vi "SCTL Sector Accumulation V2.vi"() -> (3 "New Data?":bool)   [LabVIEW 2013]
uses:
  <vilib>/rvi/Memory/Memory_Emulation/niFpgaMemoryEmulationReadFromVariant.vi
  <vilib>/rvi/Emulation/niFpgaSctlEmulationGetInTimedLoop.vi
  <vilib>/rvi/Memory/Memory_Emulation/niFpgaMemoryEmulationWriteToVariant.vi
  <vilib>/rvi/DataTransferAndStorage/Container/Common/niFpgaContainerGetUniqueNameForEmu.vi
  <vilib>/rvi/FIFO/Fifo_Resource/nirvififoEmulationSetSize.vi
  <vilib>/rvi/Emulation/niFpgaSctlEmulationFifoFullMgr.vi
  <vilib>/rvi/errors/niFpgaSetErrorForExecOnDevCompSimple.vi
  <vilib>/rvi/eio/common/nirviEmuReportErrorAndStop.vi
  <vilib>/rvi/Emulation/niFpgaSctlEmulationResourceMgr.vi
  <vilib>/rvi/Memory/Memory_Emulation/nirvimemoryFastEmulation.vi
  <vilib>/rvi/Memory/Memory_Emulation/nirvimemoryEmulation.vi
  <vilib>/rvi/DataTransferAndStorage/Container/XNode/niFpgaContainer.xnode
  <vilib>/rvi/FIFO/Fifo_Resource/nirvififoEmulationRead.vi
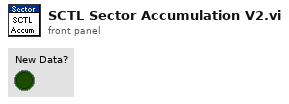
[diagram p1: front panel]
types:
  T1 = cluster{"Accumulated Intensity":u32, "Count":u16}
  T2 = cluster{"Accumulated Intensity":u32, "Count":u16}[]
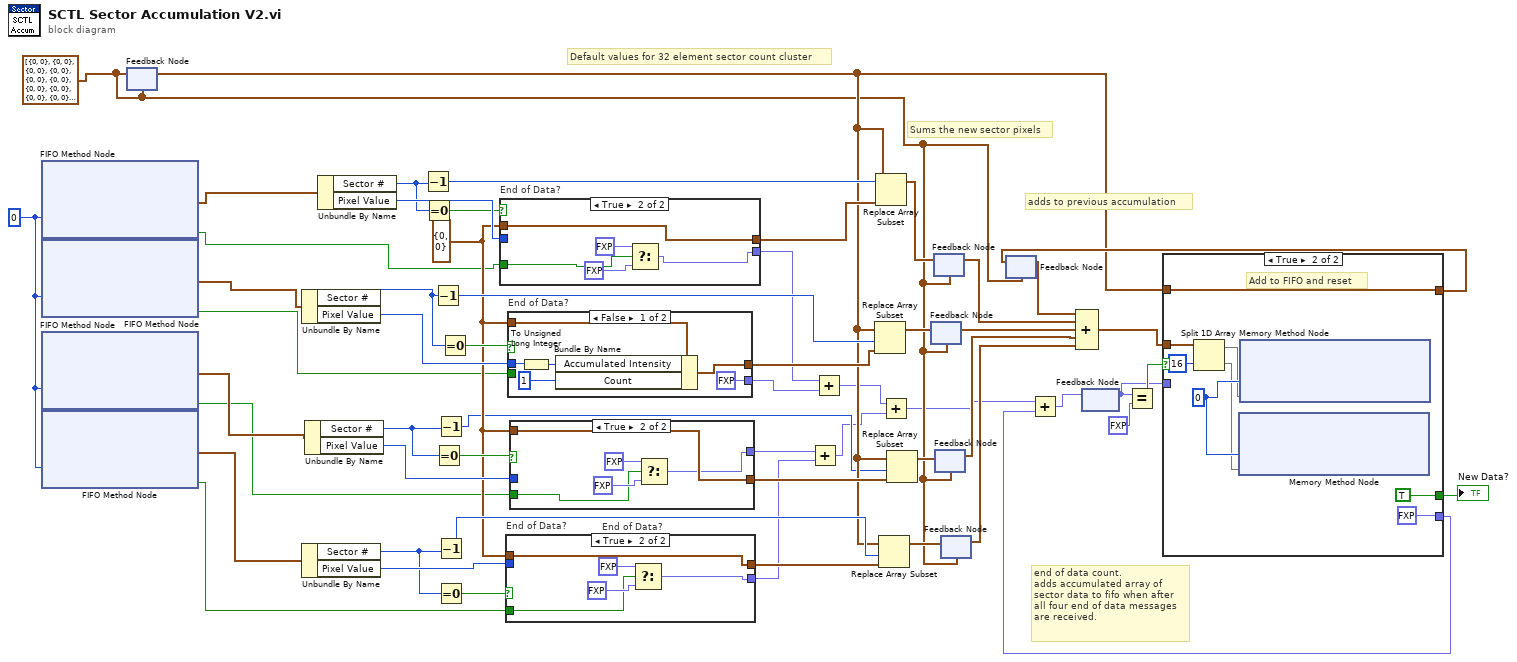
[diagram p0: block diagram]
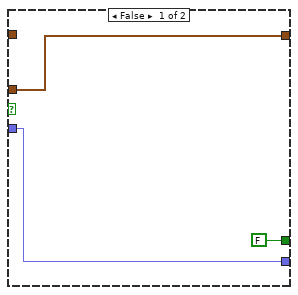
[diagram p2: hidden frame]
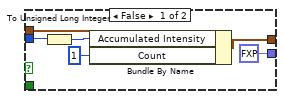
[diagram p3: hidden frame]
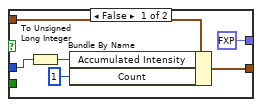
[diagram p4: hidden frame]
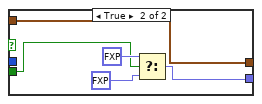
[diagram p5: hidden frame]
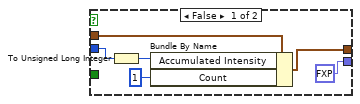
[diagram p6: hidden frame]
diagram:
  w32 = T1 {"Accumulated Intensity"=0, "Count"=0} ("Accumulated Sector Cluster")
  w10 = T2 [{"Accumulated Intensity"=0, "Count"=0}, {"Accumulated Intensity"=0, "Count"=0}, {"Accumulated Intensity"=0, "Count"=0}, {"Accumulated Intensity"=0, "Count"=0}, {"Accumulated Intensity"=0, "Count"=0}, {"Accumulated Intensity"=0, "Count"=0}, {"Accumulated Intensity"=0, "Count"=0}, {"Accumulated Intensity"=0, "Count"=0}, {"Accumulated Intensity"=0, "Count"=0}, {"Accumulated Intensity"=0, "Count"=0}, {"Accumulated Intensity"=0, "Count"=0}, {"Accumulated Intensity"=0, "Count"=0}, {"Accumulated Intensity"=0, "Count"=0}, {"Accumulated Intensity"=0, "Count"=0}, {"Accumulated Intensity"=0, "Count"=0}, {"Accumulated Intensity"=0, "Count"=0}, {"Accumulated Intensity"=0, "Count"=0}, {"Accumulated Intensity"=0, "Count"=0}, {"Accumulated Intensity"=0, "Count"=0}, {"Accumulated Intensity"=0, "Count"=0}, {"Accumulated Intensity"=0, "Count"=0}, {"Accumulated Intensity"=0, "Count"=0}, {"Accumulated Intensity"=0, "Count"=0}, {"Accumulated Intensity"=0, "Count"=0}, {"Accumulated Intensity"=0, "Count"=0}, {"Accumulated Intensity"=0, "Count"=0}, {"Accumulated Intensity"=0, "Count"=0}, {"Accumulated Intensity"=0, "Count"=0}, {"Accumulated Intensity"=0, "Count"=0}, {"Accumulated Intensity"=0, "Count"=0}, {"Accumulated Intensity"=0, "Count"=0}, {"Accumulated Intensity"=0, "Count"=0}] ("Data")
  w56 = 0 ("Timeout")
  # "end of data count.\nadds accumulated array of\nsector data to fifo when after\nall four end of data messages\nare received."
  # "adds to previous accumulation"
  # "Sums the new sector pixels"
  # "Default values for 32 element sector count cluster"
  n1 = xnode ("FIFO Method Node")("Timeout"=w56) -> ("Element"=w26:cluster{"Sector #":u8, "Pixel Value":u8}, "Timed Out?"=w22:bool)  [unwired: 1 in, 1 out]
  n2 = xnode ("FIFO Method Node")("Timeout"=w56) -> ("Element"=w25:cluster{"Sector #":u8, "Pixel Value":u8}, "Timed Out?"=w21:bool)  [unwired: 1 in, 1 out]
  n3 = xnode ("FIFO Method Node")("Timeout"=w56) -> ("Element"=w24:cluster{"Sector #":u8, "Pixel Value":u8}, "Timed Out?"=w20:bool)  [unwired: 1 in, 1 out]
  n4 = xnode ("FIFO Method Node")("Timeout"=w56) -> ("Element"=w23:cluster{"Sector #":u8, "Pixel Value":u8}, "Timed Out?"=w19:bool)  [unwired: 1 in, 1 out]
  n5 = feedback #1(w10) -> (w31:T2)
  n6 = feedback-in #1(w10) -> ()
  n7 = Unbundle By Name(w25) -> ("Sector #"=w42:u8, "Pixel Value"=w52:u8)
  n8 = Unbundle By Name(w23) -> ("Sector #"=w38:u8, "Pixel Value"=w46:u8)
  n9 = Unbundle By Name(w24) -> ("Sector #"=w40:u8, "Pixel Value"=w49:u8)
  n10 = Unbundle By Name(w26) -> ("Sector #"=w44:u8, "Pixel Value"=w54:u8)
  n11 = Decrement(x=w44) -> (x-1=w55:u8)
  n12 = Equal To 0?(x=w44) -> (x = 0?=w43:bool)
  n13 = Decrement(x=w42) -> (x-1=w51:u8)
  n14 = Equal To 0?(x=w40) -> (x = 0?=w39:bool)
  n15 = Decrement(x=w40) -> (x-1=w29:u8)
  n16 = Decrement(x=w38) -> (x-1=w48:u8)
  n17 = Equal To 0?(x=w38) -> (x = 0?=w37:bool)
  n18 = Equal To 0?(x=w42) -> (x = 0?=w41:bool)
  n19 = case "End of Data?" shown="True" w43 {
    tunnel: w54 -> [w58 _]
    tunnel: [w62 w67] -> w53
    tunnel: w32 -> [w61 w67]
    tunnel: [fxp<+,1,1> 0.0 w63] -> w9
    tunnel: w22 -> [_ w66]
    frame False {
      n20 = To Unsigned Long Integer(number=w58) -> (unsigned 32bit integer=w57:u32)
      n21 = Bundle By Name(cluster=w61, "Accumulated Intensity"=w57, "Count"=u16 1) -> (w62:T1)
    }
    frame True {
      n22 = Select(t=fxp<+,1,1> 0.0, s=w66, f=fxp<+,1,1> 0.0) -> (s? t:f=w63:fxp<+,1,1>)
    }
  }
  n23 = case "End of Data?" shown="True" w37 {
    tunnel: [w73 w78] -> w47
    tunnel: w32 -> [w72 w78]
    tunnel: w46 -> [w69 _]
    tunnel: [fxp<+,1,1> 0.0 w74] -> w6
    tunnel: w19 -> [_ w75]
    frame False {
      n24 = To Unsigned Long Integer(number=w69) -> (unsigned 32bit integer=w68:u32)
      n25 = Bundle By Name(cluster=w72, "Accumulated Intensity"=w68, "Count"=u16 1) -> (w73:T1)
    }
    frame True {
      n26 = Select(t=fxp<+,1,1> 0.0, s=w75, f=fxp<+,1,1> 1.0) -> (s? t:f=w74:fxp<+,1,1>)
    }
  }
  n27 = case "End of Data?" shown="False" w41 {
    tunnel: w52 -> [w80 _]
    tunnel: w32 -> [w84 w89]
    tunnel: [w83 w89] -> w45
    tunnel: [fxp<+,1,1> 0.0 w85] -> w8
    tunnel: w21 -> [_ w86]
    frame False {
      n28 = To Unsigned Long Integer(number=w80) -> (unsigned 32bit integer=w79:u32)
      n29 = Bundle By Name(cluster=w84, "Accumulated Intensity"=w79, "Count"=u16 1) -> (w83:T1)
    }
    frame True {
      n30 = Select(t=fxp<+,1,1> 0.0, s=w86, f=fxp<+,1,1> 1.0) -> (s? t:f=w85:fxp<+,1,1>)
    }
  }
  n31 = case "End of Data?" shown="True" w39 {
    tunnel: [w95 w100] -> w50
    tunnel: w49 -> [w91 _]
    tunnel: w32 -> [w94 w100]
    tunnel: [fxp<+,1,1> 0.0 w96] -> w7
    tunnel: w20 -> [_ w97]
    frame False {
      n32 = To Unsigned Long Integer(number=w91) -> (unsigned 32bit integer=w90:u32)
      n33 = Bundle By Name(cluster=w94, "Accumulated Intensity"=w90, "Count"=u16 1) -> (w95:T1)
    }
    frame True {
      n34 = Select(t=fxp<+,1,1> 0.0, s=w97, f=fxp<+,1,1> 1.0) -> (s? t:f=w96:fxp<+,1,1>)
    }
  }
  n35 = Add(x=w7, y=w6) -> (x+y=w4:fxp<+,2,2>)
  n36 = Add(x=w9, y=w8) -> (x+y=w5:fxp<+,2,2>)
  n37 = Replace Array Subset(array=w31, new element=w45, index=w51) -> (w16:T2)
  n38 = Replace Array Subset(array=w31, new element=w53, index=w55) -> (w18:T2)
  n39 = Replace Array Subset(array=w31, new element=w47, index=w48) -> (w12:T2)
  n40 = Add(x=w5, y=w4) -> (x+y=w3:fxp<+,3,3>)
  n41 = Replace Array Subset(array=w31, new element=w50, index=w29) -> (w15:T2)
  n42 = feedback #2(w10) -> (w14:T2)
  n43 = feedback-in #2(w16) -> ()
  n44 = feedback #3(w10) -> (w17:T2)
  n45 = feedback-in #3(w18) -> ()
  n46 = feedback #4(w10) -> (w13:T2)
  n47 = feedback-in #4(w15) -> ()
  n48 = feedback #5(w10) -> (w11:T2)
  n49 = feedback-in #5(w12) -> ()
  n50 = feedback #6(w10) -> (w28:T2)
  n51 = Compound Arithmetic op=ADD(w28, w17, w14, w13, w11) -> (w27:T2)
  n52 = feedback #7() -> (w34:fxp<+,3,3>)  [unwired: 1 in]
  n53 = Equal?(x=w34, y=fxp<+,3,3> 4.0) -> (x = y?=w35:bool)
  n54 = case shown="True" w35 {
    tunnel: w27 -> [w103 w108]
    tunnel: [w101 fxp<+,3,3> 0.0] -> w2
    tunnel: w34 -> [w101 _]
    tunnel: [w103 w110] -> w33
    tunnel: w31 -> [_ w110]
    tunnel: [FALSE ("New Data?") TRUE ("New Data?")] -> w30
    frame False {
    }
    frame True {
      w109 = 0 ("Timeout")
      # "Add to FIFO and reset"
      n55 = Split 1D Array(array=w108, index=16) -> (first subarray=w106:T2, second subarray=w105:T2)
      n56 = xnode ("Memory Method Node")("Address"=w109, "Data"=w105) -> ()  [unwired: 1 in, 1 out]
      n57 = xnode ("Memory Method Node")("Address"=w109, "Data"=w106) -> ()  [unwired: 1 in, 1 out]
    }
  }
  "New Data?" <- w30
  n58 = feedback-in #6(w33) -> ()
  n59 = Add(x=w3, y=w2) -> (x+y=w1:fxp<+,3,3>)
  n60 = feedback-in #7(w1) -> ()
